vi "angset.vi"(9 "psi":dbl, 10 "theta":dbl, 11 "phi":dbl) -> (1 "psio":dbl, 2 "thetao":dbl, 3 "phio":dbl)   [LabVIEW 2015]
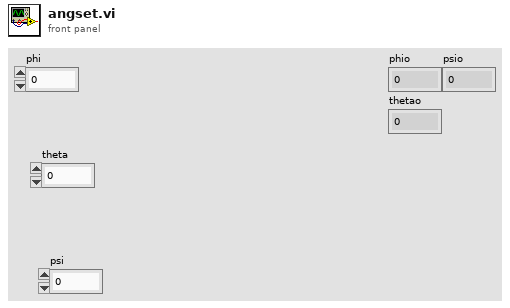
[diagram p1: front panel]
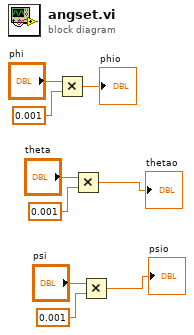
[diagram p0: block diagram]
diagram:
  n1 = Multiply ("Multiply 2")(x="phi", y=0.001) -> (x*y=→"phio":dbl)
  n2 = Multiply ("Multiply 2")(x="theta", y=0.001) -> (x*y=→"thetao":dbl)
  n3 = Multiply ("Multiply 2")(x="psi", y=0.001) -> (x*y=→"psio":dbl)
